vi "Traffic light.vi"() -> ()   [LabVIEW 2011]
panel:
  in  "Cross button":bool
  out "Boolean 3":bool
  out "Boolean 2":bool
  out "Boolean":bool
  in  "stop":bool
  out "Numeric":dbl
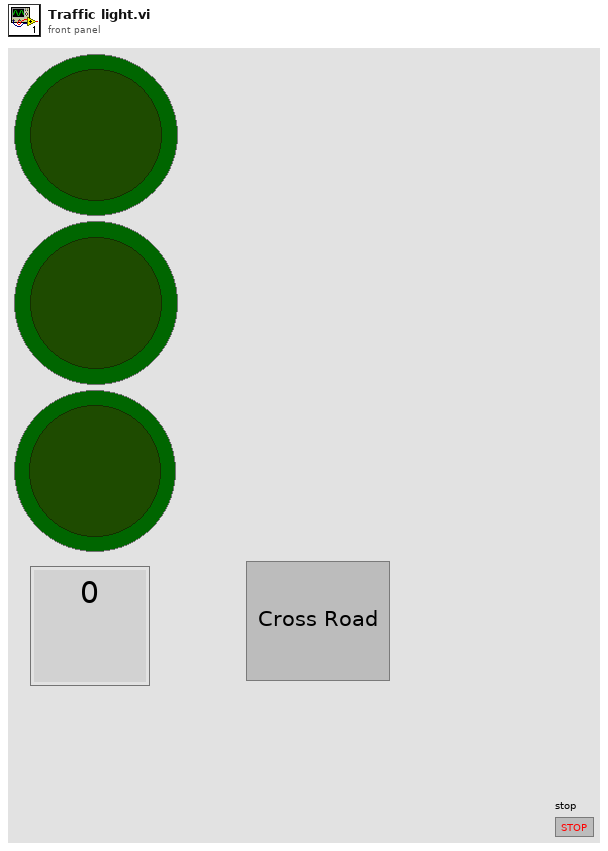
[diagram p1: front panel]
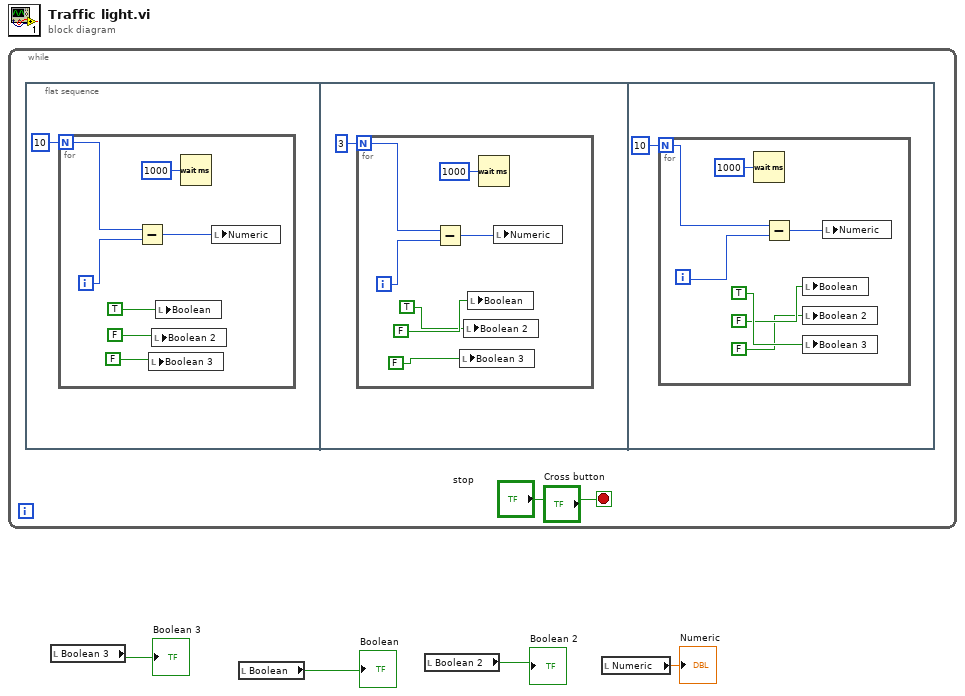
[diagram p0: block diagram]
diagram:
  n1 = while {
    stop <- "stop" stop-if-true
    n2 = flat-sequence {
      frame #0 {
        n3 = for {
          N: 10 -> [w13]
          i -> [w12]
          n4 = Subtract(x=w13, y=w12) -> (x-y=w8:i32)
          n5 = local write "Boolean 3"(FALSE) -> ()
          n6 = local write "Boolean 2"(FALSE) -> ()
          n7 = local write "Boolean"(TRUE) -> ()
          n8 = Wait (ms)(milliseconds to wait=u32 1000) -> ()  [unwired: 1 out]
          n9 = local write "Numeric"(w8) -> ()
        }
      }
      frame #1 {
        n10 = for {
          N: 3 -> [w21]
          i -> [w20]
          n11 = Subtract(x=w21, y=w20) -> (x-y=w16:i32)
          n12 = local write "Boolean 3"(FALSE) -> ()
          n13 = local write "Boolean 2"(TRUE) -> ()
          n14 = local write "Boolean"(FALSE) -> ()
          n15 = Wait (ms)(milliseconds to wait=u32 1000) -> ()  [unwired: 1 out]
          n16 = local write "Numeric"(w16) -> ()
        }
      }
      frame #2 {
        n17 = for {
          N: 10 -> [w27]
          i -> [w26]
          n18 = Wait (ms)(milliseconds to wait=u32 1000) -> ()  [unwired: 1 out]
          n19 = Subtract(x=w27, y=w26) -> (x-y=w28:i32)
          n20 = local write "Boolean"(FALSE) -> ()
          n21 = local write "Boolean 2"(FALSE) -> ()
          n22 = local write "Boolean 3"(TRUE) -> ()
          n23 = local write "Numeric"(w28) -> ()
        }
      }
    }
  }
  n24 = local read "Boolean 3"() -> (→"Boolean 3":bool)
  n25 = local read "Boolean"() -> (→"Boolean":bool)
  n26 = local read "Boolean 2"() -> (→"Boolean 2":bool)
  n27 = local read "Numeric"() -> (→"Numeric":dbl)
